vi "Native POST.vi"() -> ()   [LabVIEW 2017]
uses:
  Types/Result Configuration.ctl
  <vilib>/httpClient/POSTBuffer.vi
  <vilib>/httpClient/LabVIEWHTTPClient.lvlib
panel:
  out "error out":errorcluster
  out "Returned body":string
  out "Returned headers":string
  in  "Base URL":string="http://localhost:3000/results"
  in  "POST data":T1
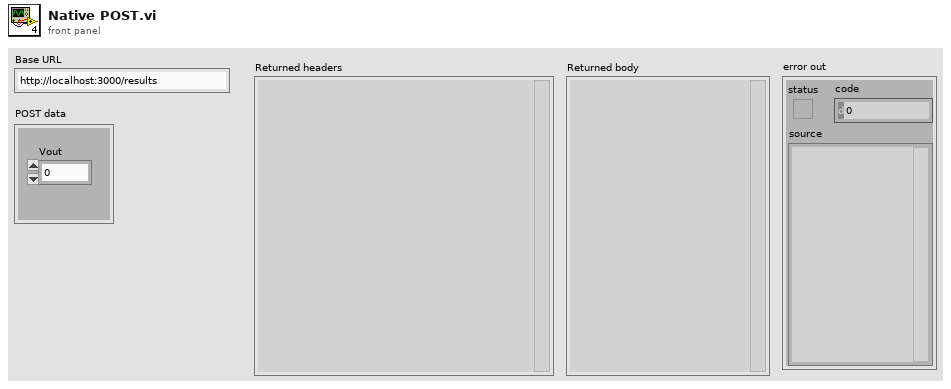
[diagram p1: front panel]
types:
  T1 = typedef "Result Configuration.ctl" = cluster{"Vout":dbl}
  T2 = typedef "LabVIEWHTTPClient.lvlib/ClientHandle.ctl" = refnum<k1>
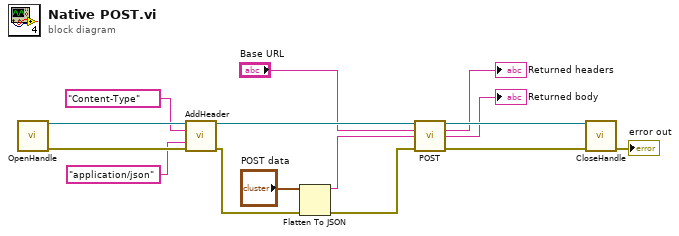
[diagram p0: block diagram]
diagram:
  n1 = call <vilib>:"OpenHandle.vi"() -> ("client handle out"=w15:T2, "error out"=w14:errorcluster)  [unwired: 14 in]
  n2 = call <vilib>:"AddHeader.vi"("client handle"=w15, "header"="Content-Type", "value"="application/json", "error in (no error)"=w14) -> ("client handle out"=w9:T2, "error out"=w10:errorcluster)  [unwired: 10 in]
  n3 = Flatten To JSON(anything="POST data", error in (no error)=w10) -> (JSON string=w6:string, 11:w8:errorcluster)  [unwired: 1 in]
  n4 = call-poly <vilib>:"POST.vi"("client handle"=w9, "url"="Base URL", "buffer"=w6, "error in (no error)"=w8) -> ("client handle out"=w5:T2, "headers"=→"Returned headers":string, "body"=→"Returned body":string, "error out"=w4:errorcluster)  [unwired: 8 in]
  n5 = call <vilib>:"CloseHandle.vi"("client handle"=w5, "error in (no error)"=w4) -> ("error out"=→"error out":errorcluster)  [unwired: 13 in]
